vi "readInXMLNative.vi"(8 "error in (no error)":errorcluster, 10 "scriptEventXML":refnum<k20>, 11 "ScriptEvent in":refnum<class "ScriptEvent.lvclass">) -> (0 "error out":errorcluster, 3 "ScriptEvent out":refnum<class "ScriptEvent.lvclass">)   [LabVIEW 2011, in "Tools.lvlib" / "Scripting.lvlib" / "ScriptEvent.lvclass"]
uses:
  ScriptEvent.lvclass
  <vilib>/xml/Close Reference(Node).vi
  <vilib>/xml/NI_XML.lvlib
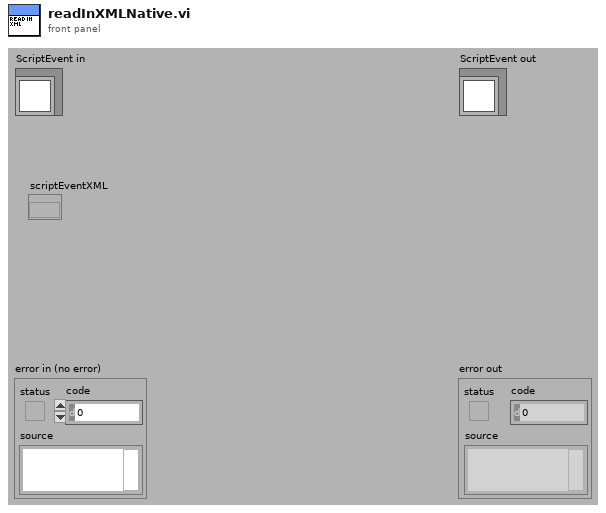
[diagram p1: front panel]
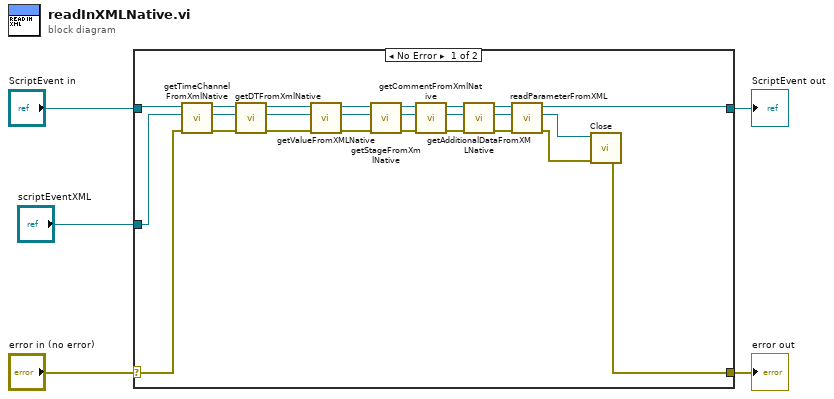
[diagram p0: block diagram]
diagram:
  n1 = case shown="No Error" "error in (no error)" {
    selector: "error in (no error)" -> [w13 w32]
    tunnel: [w12 w32] -> w4
    tunnel: [w7 w31] -> w2
    tunnel: "ScriptEvent in" -> [w30 w31]
    tunnel: "scriptEventXML" -> [w29 _]
    frame No Error {
      n2 = call "getTimeChannelFromXmlNative.vi"("error in (no error)"=w13, "eventXML"=w29, "ScriptEvent in"=w30) -> ("error out"=w27:errorcluster, "eventXML out"=w17:refnum<k20>, "ScriptEvent out"=w28:refnum<class "ScriptEvent.lvclass">)  [unwired: 6 in]
      n3 = call "getDTFromXmlNative.vi"("error in (no error)"=w27, "eventXML"=w17, "ScriptEvent in"=w28) -> ("error out"=w19:errorcluster, "eventXML out"=w18:refnum<k20>, "ScriptEvent out"=w26:refnum<class "ScriptEvent.lvclass">)  [unwired: 6 in]
      n4 = call-dynamic "getValueFromXMLNative.vi"("error in (no error)"=w19, "eventXML"=w18, "ScriptEvent in"=w26) -> ("error out"=w20:errorcluster, "eventXML out"=w14:refnum<k20>, "ScriptEvent out"=w25:refnum<class "ScriptEvent.lvclass">)  [unwired: 6 in]
      n5 = call "getStageFromXmlNative.vi"("error in (no error)"=w20, "eventXML"=w14, "ScriptEvent in"=w25) -> ("error out"=w21:errorcluster, "eventXML out"=w16:refnum<k20>, "ScriptEvent out"=w24:refnum<class "ScriptEvent.lvclass">)  [unwired: 6 in]
      n6 = call "getCommentFromXmlNative.vi"("error in (no error)"=w21, "eventXML"=w16, "ScriptEvent in"=w24) -> ("error out"=w22:errorcluster, "eventXML out"=w15:refnum<k20>, "ScriptEvent out"=w23:refnum<class "ScriptEvent.lvclass">)  [unwired: 6 in]
      n7 = call-dynamic "getAdditionalDataFromXMLNative.vi"("error in (no error)"=w22, "eventXML"=w15, "ScriptEvent in"=w23) -> ("error out"=w9:errorcluster, "eventXML out"=w10:refnum<k20>, "ScriptEvent out"=w11:refnum<class "ScriptEvent.lvclass">)  [unwired: 6 in]
      n8 = call-dynamic "readParameterFromXML.vi"("error in (no error)"=w9, "eventXML"=w10, "ScriptEvent in"=w11) -> ("error out"=w6:errorcluster, "eventXML out"=w8:refnum<k20>, "ScriptEvent out"=w7:refnum<class "ScriptEvent.lvclass">)  [unwired: 6 in]
      n9 = call-poly <vilib>:"Close.vi"("error in (no error)"=w6, "node"=w8) -> ("error out"=w12:errorcluster)  [unwired: 7 in]
    }
    frame Error {
    }
  }
  "error out" <- w4
  "ScriptEvent out" <- w2
